vi "To Unicode String_DK.vi"(3 "error in":errorcluster, 4 "Big Endian?":bool, 5 "Code Page":i32(ring) items=["System default"=0, "Latin-1"=1252, "Japanese"=932, "Korean"=947, "Chinese simplified"=936, "Chinese traditional"=950, "Central Europe"=1250, "Cyrillic"=1251, "Greek"=1253, "Turkish"=1254, "Hebrew"=1255, "Arabic"=1256, "Baltic"=1257, "Thai"=874, "Vietnamese"=783, "UTF8"=65001, "UTF-7"=65000], 6 "Multibyte String":string="tété") -> (0 "error out":errorcluster, 2 "Unicode string":string)   [LabVIEW 2024]
uses:
  kernel32.dll
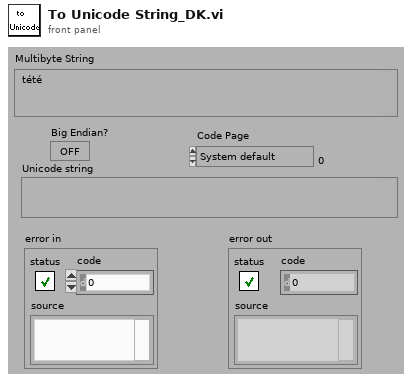
[diagram p1: front panel]
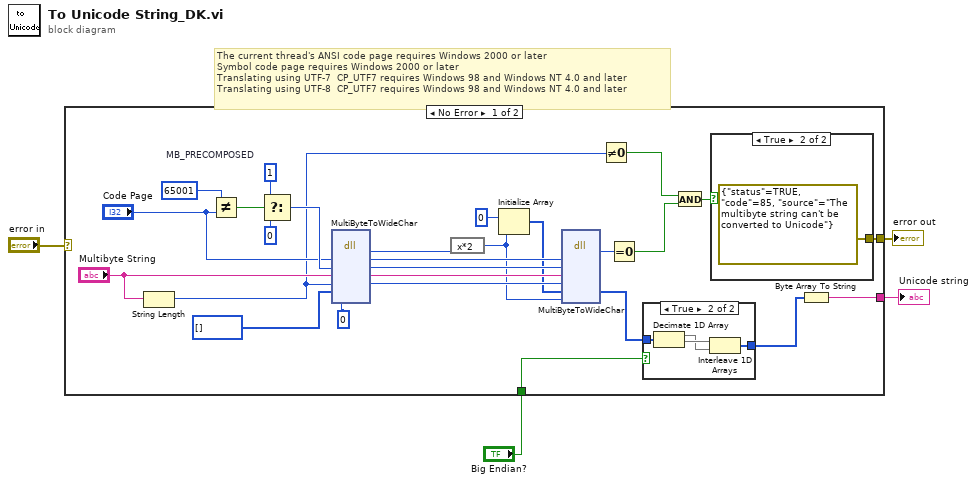
[diagram p0: block diagram]
diagram:
  # "The current thread's ANSI code page requires Windows 2000 or later\nSymbol code page requires Windows 2000 or later\nTranslating using UTF-7  CP_UTF7 requires Windows 98 and Windows NT 4.0 and later\nTranslating using UTF-8  CP_UTF7 requires Windows 98 and Windows NT 4.0 and later"
  n1 = case shown="No Error" "error in" {
    selector: "error in" -> [_ w38]
    tunnel: [w13 _] -> w4
    tunnel: [w7 w38] -> w2
    tunnel: "Big Endian?" -> [w5 _]
    frame No Error {
      w17 = u32 1  # MB_PRECOMPOSED
      n2 = String Length(string="Multibyte String") -> (length=w11:i32)
      n3 = Not Equal?(x=u32 65001, y="Code Page") -> (x != y?=w19:bool)
      n4 = Select(t=w17, s=w19, f=u32 0) -> (s? t:f=w18:u32)
      n5 = dll-call lib="Kernel32.DLL" fn="MultiByteToWideChar"("Codepage"="Code Page", "dwFlags"=w18, "lpStringA"="Multibyte String", "StringSize"=w11, "lpStringW"=u8[] [], "buffersize"=0) -> (w27:i32, "Codepage"=w26:u32, "dwFlags"=w25:u32, "lpStringA"=w24:string, "StringSize"=w23:i32)  [unwired: 5 in, 2 out]
      n6 = expression code="x*2"(w27) -> (w21:i32)
      n7 = Initialize Array(u8 0, w21) -> (w22:u8[])
      n8 = dll-call lib="Kernel32.DLL" fn="MultiByteToWideChar"("Codepage"=w26, "dwFlags"=w25, "lpStringA"=w24, "StringSize"=w23, "lpStringW"=w22, "buffersize"=w21) -> (w12:i32, "lpStringW"=w15:u8[])  [unwired: 8 in, 2 out]
      n9 = Not Equal To 0?(x=w11) -> (x != 0?=w9:bool)
      n10 = Equal To 0?(x=w12) -> (x = 0?=w10:bool)
      n11 = case shown="True" w5 {
        tunnel: w15 -> [w32 w34]
        tunnel: [w32 w33] -> w6
        frame False {
        }
        frame True {
          n12 = Decimate 1D Array(w34) -> (w35:u8[], w36:u8[])
          n13 = Interleave 1D Arrays(w36, w35) -> (w33:u8[])
        }
      }
      n14 = And(x=w9, y=w10) -> (x .and. y?=w8:bool)
      n15 = case shown="True" w8 {
        tunnel: [_ errorcluster {"status"=TRUE, "code"=85, "source"="The multibyte string can't be converted to Unicode"} ("error IO")] -> w7
        frame False {
        }
        frame True {
        }
      }
      n16 = Byte Array To String(unsigned byte array=w6) -> (string=w13:string)
    }
    frame Error {
    }
  }
  "Unicode string" <- w4
  "error out" <- w2
